vi "get_ratio.vi"(8 "error in (no error)":errorcluster, 11 "TrajectoryDL090201FrameScan in":refnum<class "TrajectoryDL090201FrameScan.lvclass">) -> (0 "error out":errorcluster, 1 "y":dbl, 2 "x":dbl, 3 "TrajectoryDL090201FrameScan out":refnum<class "TrajectoryDL090201FrameScan.lvclass">, 4 "y normalised":dbl, 6 "x normalised":dbl)   [LabVIEW 2010, in "TrajectoryDL090201FrameScan.lvclass"]
uses:
  TrajectoryDL090201FrameScan.lvclass
  TrajectoryDL090201FrameScan.lvclass/TrajectoryDL090201FrameScan.ctl
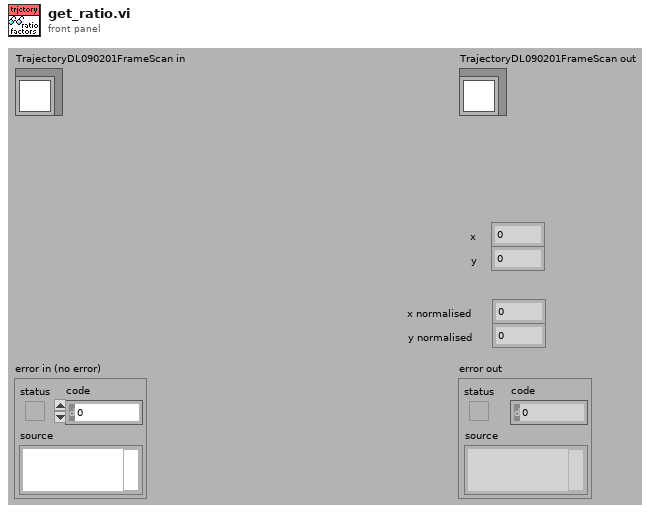
[diagram p1: front panel]
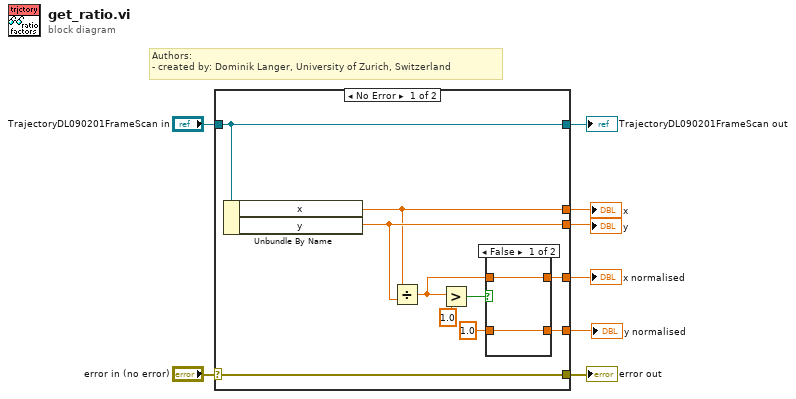
[diagram p0: block diagram]
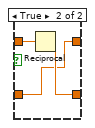
[diagram p2: hidden frame]
diagram:
  # "Authors: \n- created by: Dominik Langer, University of Zurich, Switzerland"
  n1 = case shown="No Error" "error in (no error)" {
    selector: "error in (no error)" -> [w18 w24]
    tunnel: [w18 w24] -> w7
    tunnel: [w17 w25] -> w5
    tunnel: "TrajectoryDL090201FrameScan in" -> [w17 w25]
    tunnel: [w15 _] -> w4
    tunnel: [w16 _] -> w3
    tunnel: [w10 _] -> w2
    tunnel: [w9 _] -> w1
    frame No Error {
      n2 = Unbundle By Name(w17) -> ("x"=w15:dbl, "y"=w16:dbl)
      n3 = Divide(x=w15, y=w16) -> (x/y=w12:dbl)
      n4 = Greater?(x=w12, y=1.0) -> (0:w13:bool)
      n5 = case shown="False" w13 {
        tunnel: [w20 w21] -> w10
        tunnel: w12 -> [w20 w23]
        tunnel: [w19 w22] -> w9
        tunnel: 1.0 ("y") -> [w19 w21]
        frame False {
        }
        frame True {
          n6 = Reciprocal(x=w23) -> (1/x=w22:dbl)
        }
      }
    }
    frame Error {
    }
  }
  "error out" <- w7
  "TrajectoryDL090201FrameScan out" <- w5
  "x" <- w4
  "y" <- w3
  "x normalised" <- w2
  "y normalised" <- w1
